vi "NI VeriStand - Set Custom Device Channel Type.vi"(8 "error in (no error)":errorcluster, 10 "Type":T1, 11 "Channel Ref in":T2 format="%.0x") -> (0 "error out":errorcluster, 3 "Channel Ref out":T2=18446744073709551615 format="%.0x")   [LabVIEW 2020, in "Custom Device API.lvlib"]
doc: "Sets whether the channel specified by <B>Channel Ref in</B> is an Input or an Output channel. Input channels receive values from the VeriStand Engine. Output channels send values to the VeriStand Engine."
uses:
  <vilib>/NI VeriStand/Custom Device API/Custom Device API.lvlib
  <vilib>/NI VeriStand/Custom Device API/Custom Device Item Ref.ctl
  <vilib>/NI VeriStand/Custom Device API/Custom Device Channel Type.ctl
  ff2e2633-3484-48f7-984c-1bb0f43d8271.vi
  <vilib>/NI VeriStand/Custom Device API/Custom Device Offline Path.vi
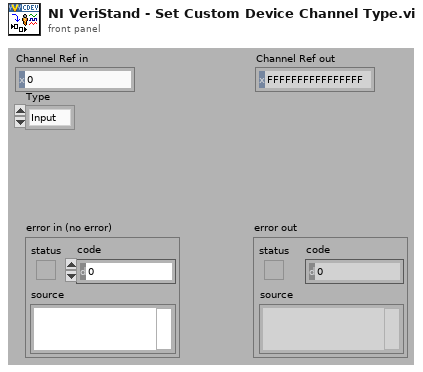
[diagram p1: front panel]
types:
  T1 = typedef "Custom Device API.lvlib/Custom Device Channel Type.ctl" = enum16{"Input", "Output"}
  T2 = typedef "Custom Device API.lvlib/Custom Device Item Ref.ctl" = u64
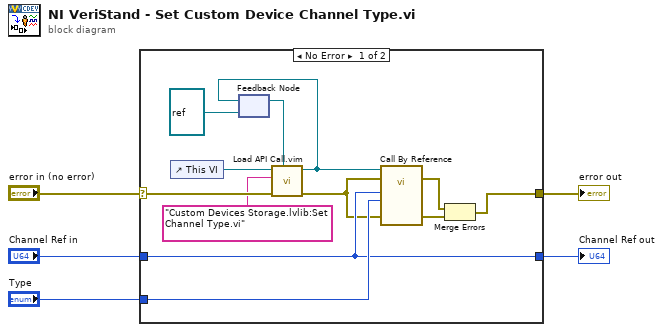
[diagram p0: block diagram]
diagram:
  n1 = case shown="No Error" "error in (no error)" {
    selector: "error in (no error)" -> [w11 w19]
    tunnel: [w16 w19] -> w5
    tunnel: "Channel Ref in" -> [w14 w18]
    tunnel: [w14 w18] -> w3
    tunnel: "Type" -> [w15 _]
    frame No Error {
      n2 = control-ref of="This VI"() -> (w12:refnum<vi>)
      n3 = feedback #1(refnum<vi> refnum ("type specifier VI Refnum (for type only)")) -> (w13:refnum<vi>)
      n4 = call "Load API Call.vim"("VI reference in"=w13, "error in (no error)"=w11, "VI qualified name"="Custom Devices Storage.lvlib:Set Channel Type.vi", "Caller VI ref"=w12) -> ("error out"=w10:errorcluster, "VI reference"=w9:refnum<vi>)  [unwired: 6 in]
      n5 = feedback-in #1(w9) -> ()
      n6 = call-by-ref "?"(reference=w9, error in=w10, 8:"error in (no error)"=w10, "Type"=w15, "Channel Ref in"=w14) -> (error out=w6:errorcluster, 0:"error out"=w17:errorcluster)  [unwired: 7 in, 2 out]
      n7 = Merge Errors(w6, w17) -> (w16:errorcluster)
    }
    frame Error {
    }
  }
  "error out" <- w5
  "Channel Ref out" <- w3
